vi "Write Startup Model-View Configuration.vi"(7 "Application Style":refnum<class "IApplicationStyle.lvclass">, 8 "Mediator Type":refnum<class "IMediator.lvclass">, 9 "Model Type":refnum<class "IModel.lvclass">, 10 "Startup View Configuration":refnum<class "IViewable.lvclass">, 11 "IViewModel In":refnum<class "IViewModel.lvclass">) -> (3 "IViewModel Out":refnum<class "IViewModel.lvclass">)   [LabVIEW 2020, in "MVA Framework.lvlib" / "IViewModel.lvlib" / "IViewModel.lvclass"]
doc: "此构造函数仅在公共调用时被弃用。它应该被可扩展的“Construct MVA Application.vim”所取代，它通过向一个或多个接收器添加可选的框架级事件日志来扩展。"
uses:
  IViewModel.lvclass
  IViewable/IViewable/IViewable.lvclass
  mva-core/Source/IModel/IModel/IModel.lvclass
  mva-core/Source/IMediator/IMediator/IMediator.lvclass
  IViewable/IApplicationStyle/IApplicationStyle.lvclass
  IViewModel.lvclass/IViewModel.ctl
  IViewManager/IViewManager Messages/Launch Nested Views Msg/Launch Nested Views Msg.lvclass/Launch Nested Views Msg.ctl
  IViewManager/IViewManager/IViewManager.lvclass/IViewManager.ctl
  IViewManager/IViewManager Messages/Launch Nested Views Msg/Launch Nested Views Msg.lvclass
  IViewManager/IViewManager/IViewManager.lvclass
panel:
  # "Replace public calls of this method with\nConstruct MVA Application.vim\n将此方法的公共调用替换为\n构建MVA应用程序.vim"
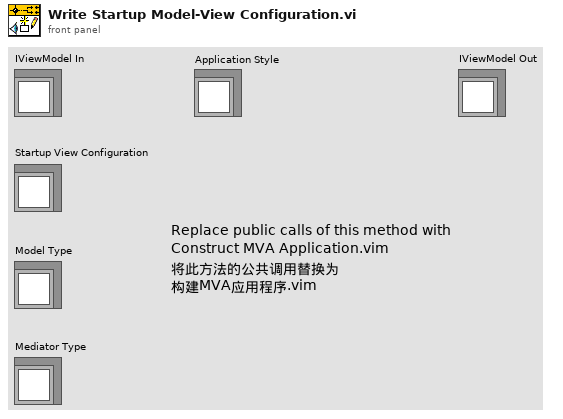
[diagram p1: front panel]
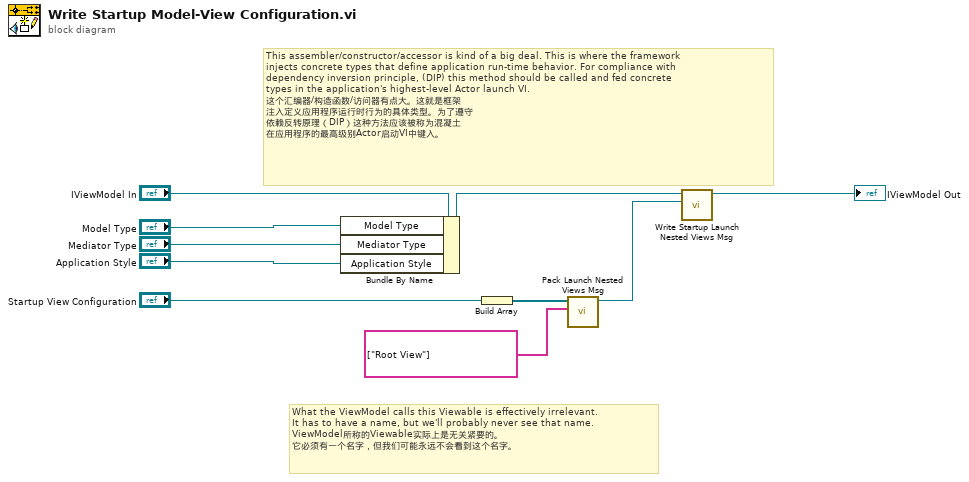
[diagram p0: block diagram]
diagram:
  # "This assembler/constructor/accessor is kind of a big deal. This is where the framework\ninjects concrete types that define application run-time behavior. For compliance with\ndependency inversion principle, (DIP) this method should be called and fed concrete\ntypes in the application's highest-level Actor launch VI.\n这个汇编器/构造函数/访问器有点大。这就是框架\n注入定义应用程序运行时行为的具体类型。为了遵守\n依赖反转原理（DIP）这种方法应该被称为混凝土\n在应用程序的最高级别Actor启动VI中键入。"
  # "What the ViewModel calls this Viewable is effectively irrelevant.\nIt has to have a name, but we'll probably never see that name.\nViewModel所称的Viewable实际上是无关紧要的。\n它必须有一个名字，但我们可能永远不会看到这个名字。"
  n1 = Bundle By Name(cluster="IViewModel In", "Model Type"="Model Type", "Mediator Type"="Mediator Type", "Application Style"="Application Style") -> (w4:refnum<class "IViewModel.lvclass">)
  n2 = Build Array("Startup View Configuration") -> (w8:refnum<class "IViewable.lvclass">[])
  n3 = call "Pack Launch Nested Views Msg.vi"("View Labels"=string[] ["Root View"] ("View Labels (optional)"), "Nested Views"=w8) -> ("Launch Nested Views Msg"=w6:refnum<class "Launch Nested Views Msg.lvclass">)  [unwired: 9 in]
  n4 = call "Write Startup Launch Nested Views Msg.vi"("Launch Nested Views Msg"=w6, "IViewManager in"=w4) -> ("IViewManager out"=→"IViewModel Out":refnum<class "IViewModel.lvclass">)  [unwired: 9 in]
